vi "store error_handler queue.vi"(8 "error in":errorcluster) -> (0 "error out":errorcluster)   [LabVIEW 2020]
uses:
  devices/devices Messages/store error_handler queue Msg/store error_handler queue Msg.lvclass/store error_handler queue Msg.ctl
  <vilib>/ActorFramework/Message Enqueuer/Message Enqueuer.lvclass/Message Enqueuer.ctl
  <vilib>/ActorFramework/Message Enqueuer/Enqueue.vi
  devices/devices Messages/store error_handler queue Msg/store error_handler queue Msg.lvclass
  C:/Program Files (x86)/National Instruments/LabVIEW 2020/vi.lib/ActorFramework/Message/Message.lvclass
  <vilib>/ActorFramework/Message Priority Queue/Priority Enqueue.vi
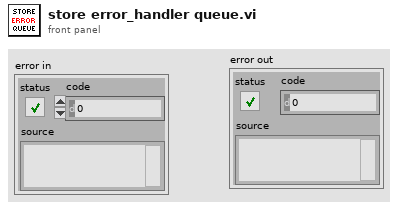
[diagram p1: front panel]
types:
  T1 = typedef "EquipmentCluster.ctl" = cluster{"Device":string, "Function":string, "Name":string, "Driver":string, "Address":string, "Device_queue":refnum<class "Message Enqueuer.lvclass">}
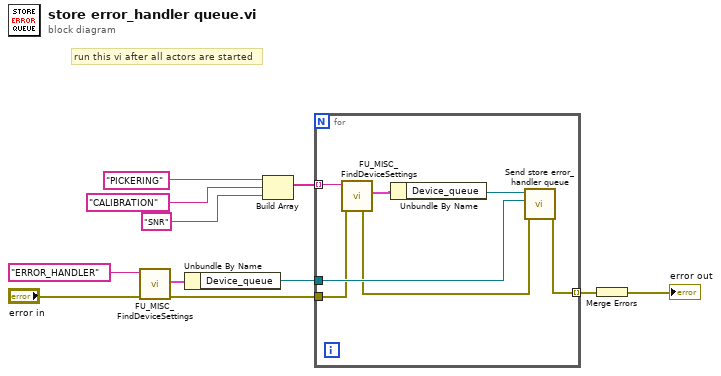
[diagram p0: block diagram]
diagram:
  # "run this vi after all actors are started"
  n1 = call "FU_MISC_FindDeviceSettings.vi"("ErrorIn"="error in", "DeviceID"="ERROR_HANDLER") -> ("ErrorOut"=w1:errorcluster, "Settings"=w7:T1)  [unwired: 7 in, 1 out]
  n2 = Unbundle By Name(w7) -> ("Device_queue"=w5:refnum<class "Message Enqueuer.lvclass">)
  n3 = Build Array("PICKERING" ("DeviceID"), "CALIBRATION" ("DeviceID"), "SNR" ("DeviceID")) -> (w11:string[])
  n4 = for {
    tunnel: w11 -> [w17] mode=indexing
    tunnel: w5 -> [w15]
    tunnel: [w14] -> w4 mode=indexing
    tunnel: w1 -> [w13]
    n5 = call "FU_MISC_FindDeviceSettings.vi"("ErrorIn"=w13, "DeviceID"=w17) -> ("ErrorOut"=w12:errorcluster, "Settings"=w18:T1)  [unwired: 7 in, 1 out]
    n6 = Unbundle By Name(w18) -> ("Device_queue"=w16:refnum<class "Message Enqueuer.lvclass">)
    n7 = call "Send store error_handler queue.vi"("error in (no error)"=w12, "error handler queue"=w15, "Message Enqueuer"=w16) -> ("error out"=w14:errorcluster)  [unwired: 7 in, 1 out]
  }
  n8 = Merge Errors(w4) -> (→"error out":errorcluster)
